vi "CMD_Shooter.vi"(1 "Line":string) -> (0 "Done":bool)   [LabVIEW 2015]
uses:
  Robot Global Data.vi
  <vilib>/Rock Robotics/Network Tables/NT Read Number.vi
  <vilib>/Rock Robotics/WPI/Utilities/WPI_GetSetVariantRefNum.vi
  AppleScript Global Data.vi
panel:
  in  "Parameters":i32[](array[numeric])=[0, 1, 0, 2]
  in  "Subcommands":string[](array[string])=["fire", "to", "align", "to"]
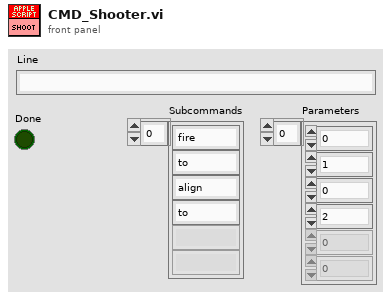
[diagram p1: front panel]
types:
  T1 = typedef "WPI_RobotDriveDevRef.ctl" = cluster{"DevStatus":errorcluster, "Motors[]":T2[], "Square Inputs":bool, "Max Output":dbl}
  T2 = typedef "WPI_MotorControlDeviceRef.ctl" = cluster{"DeviceStatus":errorcluster, "Type":T3, "PWM":cluster{"PWM Channel":T4, "DeadBand":T5}, "CAN":cluster{"Device Number":u8, "Control Mode":T6, "Semaphore":T7, "Max Vout":dbl, "TalonSRX Control Mode":T8}, "Invert":bool}
  T3 = typedef "WPI_MotorControlType.ctl" = enum16{"PWM", "CAN", "CANTalonSRX"}
  T4 = typedef "FPGA_DIOPWMChannel.ctl" = enum8{"PWM 0", "PWM 1", "PWM 2", "PWM 3", "PWM 4", "PWM 5", "PWM 6", "PWM 7", "PWM 8", "PWM 9", "PWM MXP 0", "PWM MXP 1", "PWM MXP 2", "PWM MXP 3", "PWM MXP 4", "PWM MXP 5", "PWM MXP 6", "PWM MXP 7", "PWM MXP 8", "PWM MXP 9", "Invalid"}
  T5 = typedef "WPI_PWMDeadband.ctl" = cluster{"Name":string, "maxPositivePwm":i32, "minPositivePwm":i32, "centerPwm":i32, "maxNegativePwm":i32, "minNegativePwm":i32, "angularRange":u16}
  T6 = typedef "WPI_CANJaguar_ControlMode.ctl" = enum8{"Percent VBus", "Current", "Speed", "Position", "Voltage"}
  T7 = typedef "Semaphore RefNum" = refnum<k1>
  T8 = typedef "WPI_CANTalonSRX_APIControlMode.ctl" = enum8{"Percent VBus", "Speed", "Position", "Slave", "Unchanged / Invalid", "Voltage Compensation", "Current", "Motion Profile"}
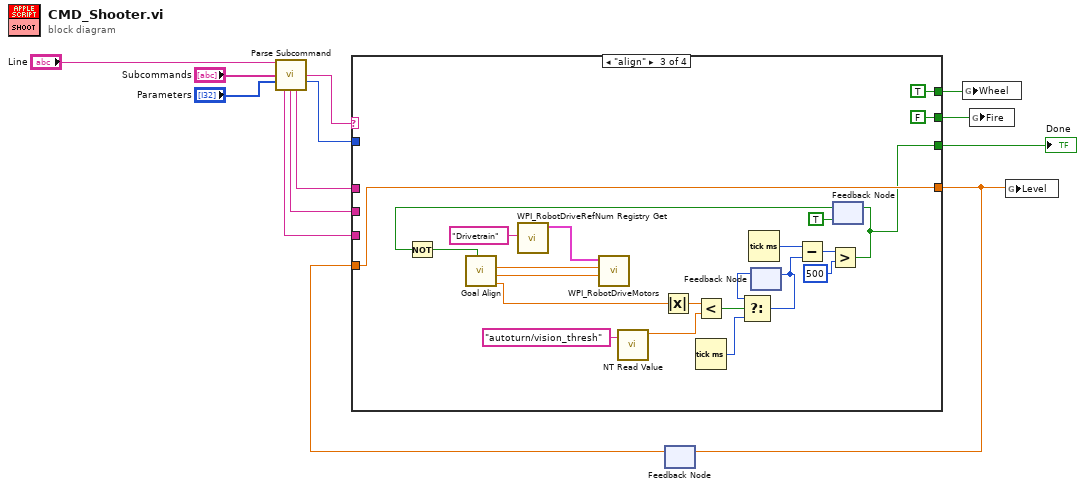
[diagram p0: block diagram]
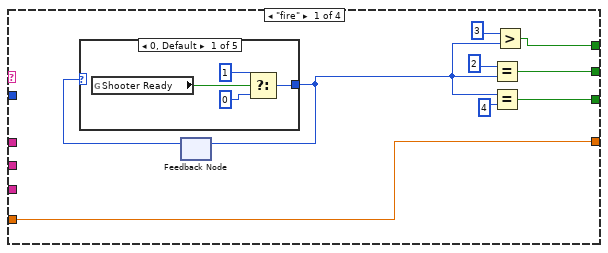
[diagram p2: hidden frame]
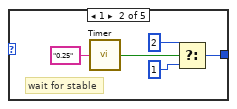
[diagram p3: hidden frame]
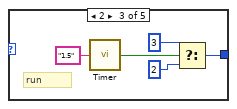
[diagram p4: hidden frame]
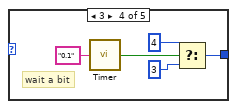
[diagram p5: hidden frame]
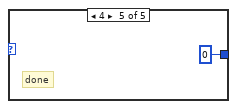
[diagram p6: hidden frame]
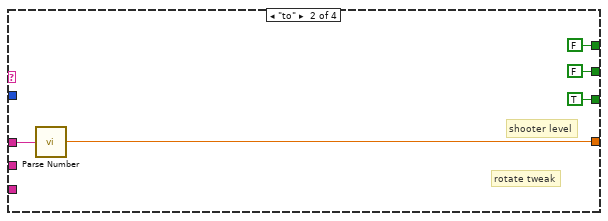
[diagram p7: hidden frame]
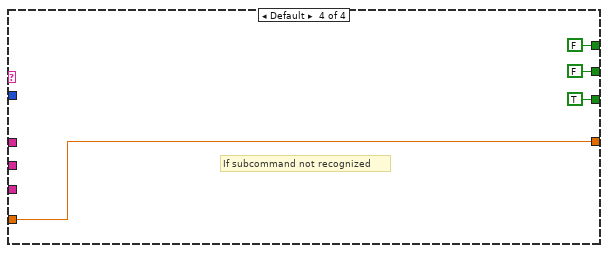
[diagram p8: hidden frame]
diagram:
  n1 = call "Parse Subcommand.vi"("Text In"="Line", "Subcommands"="Subcommands", "Parameters"="Parameters") -> ("Subcommand"=w10:string, "# of Parameters"=w9:i32, "Parameter 3"=w6:string, "Parameter 2"=w7:string, "Parameter 1"=w8:string)  [unwired: 6 in, 2 out]
  n2 = feedback #1() -> (w4:dbl)  [unwired: 1 in]
  n3 = case shown="\"align\"" w10 {
    tunnel: w9 -> [_ _ _ _]
    tunnel: w8 -> [_ w47 _ _]
    tunnel: w7 -> [_ _ _ _]
    tunnel: w6 -> [_ _ _ _]
    tunnel: [w14 TRUE w48 TRUE] -> w5
    tunnel: [w22 w43 w69 w72] -> w3
    tunnel: w4 -> [w22 _ w69 w72]
    tunnel: [w17 FALSE TRUE FALSE] -> w2
    tunnel: [w19 FALSE FALSE FALSE] -> w1
    frame "fire" {
      n4 = feedback #2() -> (w21:i32)  [unwired: 1 in]
      n5 = case shown="0, Default" w21 {
        tunnel: [w24 w29 w34 w39 0] -> w16
        frame 0, Default {
          n6 = global read "Robot Global Data.vi" "Shooter Ready"() -> (w23:bool)
          n7 = Select(t=1, s=w23, f=0) -> (s? t:f=w24:i32)
        }
        frame 1 {
          # "wait for stable"
          n8 = call "Timer.vi"("Seconds (string)"="0.25") -> ("Done"=w28:bool)
          n9 = Select(t=2, s=w28, f=1) -> (s? t:f=w29:i32)
        }
        frame 2 {
          # "run"
          n10 = call "Timer.vi"("Seconds (string)"="1.5") -> ("Done"=w33:bool)
          n11 = Select(t=3, s=w33, f=2) -> (s? t:f=w34:i32)
        }
        frame 3 {
          # "wait a bit"
          n12 = call "Timer.vi"("Seconds (string)"="0.1") -> ("Done"=w38:bool)
          n13 = Select(t=4, s=w38, f=3) -> (s? t:f=w39:i32)
        }
        frame 4 {
          # "done"
        }
      }
      n14 = feedback-in #2(w16) -> ()
      n15 = Equal?(x=2, y=w16) -> (x = y?=w19:bool)
      n16 = Equal?(x=w16, y=4) -> (x = y?=w14:bool)
      n17 = Greater?(x=3, y=w16) -> (0:w17:bool)
    }
    frame "to" {
      # "rotate tweak"
      # "shooter level"
      n18 = call "Parse Number.vi"("String"=w47) -> ("Number"=w43:dbl)
    }
    frame "align" {
      n19 = call <vilib>:"WPI_RobotDriveRefNum Registry Get.vi"("refnum name"="Drivetrain") -> ("RobotDriveDevRef"=w66:T1)  [unwired: 9 in, 1 out]
      n20 = call-poly <vilib>:"NT Read Value.vi"("Name"="autoturn/vision_thresh") -> ("Numeric"=w54:dbl)  [unwired: 9 in, 1 out]
      n21 = Tick Count (ms)() -> (millisecond timer value=w57:u32)
      n22 = Tick Count (ms)() -> (millisecond timer value=w59:u32)
      n23 = feedback #3() -> (w58:u32)  [unwired: 1 in]
      n24 = feedback #4(TRUE) -> (w51:bool)
      n25 = Not(x=w51) -> (.not. x?=w50:bool)
      n26 = call "Goal Align.vi"("last"=w50) -> ("Left"=w65:dbl, "Right"=w64:dbl, "turn err"=w52:dbl)  [unwired: 7 in]
      n27 = call <vilib>:"WPI_RobotDriveMotors.vi"("RightSpeed"=w64, "LeftSpeed"=w65, "RobotDriveDevRef"=w66) -> ()  [unwired: 6 in, 3 out]
      n28 = Absolute Value(x=w52) -> (abs(x)=w53:dbl)
      n29 = Less?(x=w53, y=w54) -> (x < y?=w56:bool)
      n30 = Select(t=w58, s=w56, f=w57) -> (s? t:f=w60:u32)
      n31 = feedback-in #3(w60) -> ()
      n32 = Subtract(x=w59, y=w60) -> (x-y=w61:u32)
      n33 = Greater?(x=w61, y=u32 500) -> (0:w48:bool)
      n34 = feedback-in #4(w48) -> ()
    }
    frame Default {
      # "If subcommand not recognized"
    }
  }
  "Done" <- w5
  n35 = feedback-in #1(w3) -> ()
  n36 = global write "AppleScript Global Data.vi" "Wheel"(w2) -> ()
  n37 = global write "AppleScript Global Data.vi" "Fire"(w1) -> ()
  n38 = global write "AppleScript Global Data.vi" "Level"(w3) -> ()
